vi "Autonomous Independent.vi"() -> ()   [LabVIEW 2012]
doc: "This VI is called when autonomous begins, and will automatically be terminated when autonomous ends. You can carry out timed or sensor driven robot movement independently without needing to return to the caller."
uses:
  <vilib>/Rock Robotics/WPI/SafetyOutput/WPI_SafetyOutputConfigMenu.ctl
  Robot Global Data.vi
  <vilib>/Rock Robotics/WPI/RobotDrive/WPI_RobotDriveGetSetRefNum.vi
  <vilib>/Rock Robotics/WPI/Joystick/WPI_JoystickGetSetRefNum.vi
  <vilib>/Rock Robotics/WPI/RobotDrive/WPI_RobotDriveArcadeDrive_Standard(NoSaturation).vi
panel:
  out "Current Movement, for debugging":T1 {"Y Joystick Value" scale=1.0..-1.0; "X Joystick Value" scale=-1.0..1.0}
  in  "Array of robot movements":T2(array[cluster]) {"Y Joystick Value" scale=1.0..-1.0; "X Joystick Value" scale=-1.0..1.0}
  # "Be sure to right-click and choose Data Operations>>Make Current Value default if you want to save the array values with the VI"
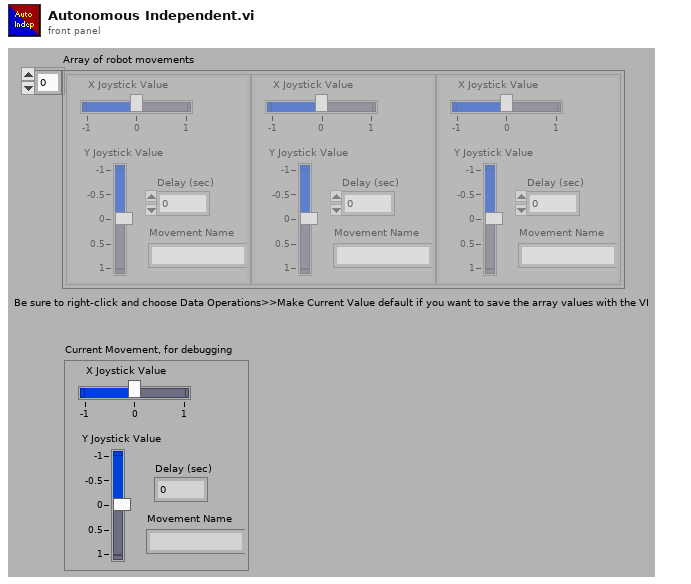
[diagram p1: front panel]
types:
  T1 = cluster{"X Joystick Value":dbl, "Y Joystick Value":dbl, "Delay (sec)":dbl, "Movement Name":string}
  T2 = cluster{"X Joystick Value":dbl, "Y Joystick Value":dbl, "Delay (sec)":dbl, "Movement Name":string}[]
  T3 = typedef "WPI_JoystickDevRef.ctl" = cluster{"Device":T4}
  T4 = typedef "WPI_JoystickDeviceEnum.ctl" = enum16{"USB 1", "USB 2", "USB 3", "USB 4", "Kinect 1", "Kinect 2"}
  T5 = cluster{"axis 1 (x)":dbl, "axis 2 (y)":dbl, "axis 3 (throttle)":dbl, "axis 4":dbl, "axis 5":dbl, "axis 6":dbl}
  T6 = typedef "WPI_SafetyOutputConfigMenu.ctl" = enum16{"Enable", "Disable"}
  T7 = typedef "WPI_RobotDriveDevRef.ctl" = cluster{"DevStatus":errorcluster, "Motors[]":T8[], "Square Inputs":bool, "Max Output":dbl, "Isochronous":bool}
  T8 = typedef "WPI_MotorControlDeviceRef.ctl" = cluster{"DeviceStatus":errorcluster, "Type":enum16{"PWM", "CAN"}, "PWM":cluster{"Digital Module":T9, "PWM Channel":T10, "DeadBand":T11}, "CAN":cluster{"Device Number":u8, "Control Mode":T12, "Semaphore":T13, "Max Vout":dbl}, "Invert":bool, "TransformRef":T14, "InvTransformRef":T14}
  T9 = typedef "FPGA_TypedefDigitalModule.ctl" = enum16{"Digital Module 1", "Digital Module 2"}
  T10 = typedef "FPGA_DIOPWMChannel.ctl" = enum8{"PWM 1", "PWM 2", "PWM 3", "PWM 4", "PWM 5", "PWM 6", "PWM 7", "PWM 8", "PWM 9", "PWM 10", "Invalid"}
  T11 = typedef "WPI_PWMDeadband.ctl" = cluster{"Name":string, "maxPositivePwm":i32, "minPositivePwm":i32, "centerPwm":i32, "maxNegativePwm":i32, "minNegativePwm":i32, "angularRange":u16}
  T12 = typedef "WPI_CANJaguar_ControlMode.ctl" = enum8{"Percent VBus", "Current", "Speed", "Position", "Voltage"}
  T13 = typedef "Semaphore RefNum" = refnum<k1>
  T14 = typedef "WPI_PWMTransform_ConPane.ctl" = refnum<vi>
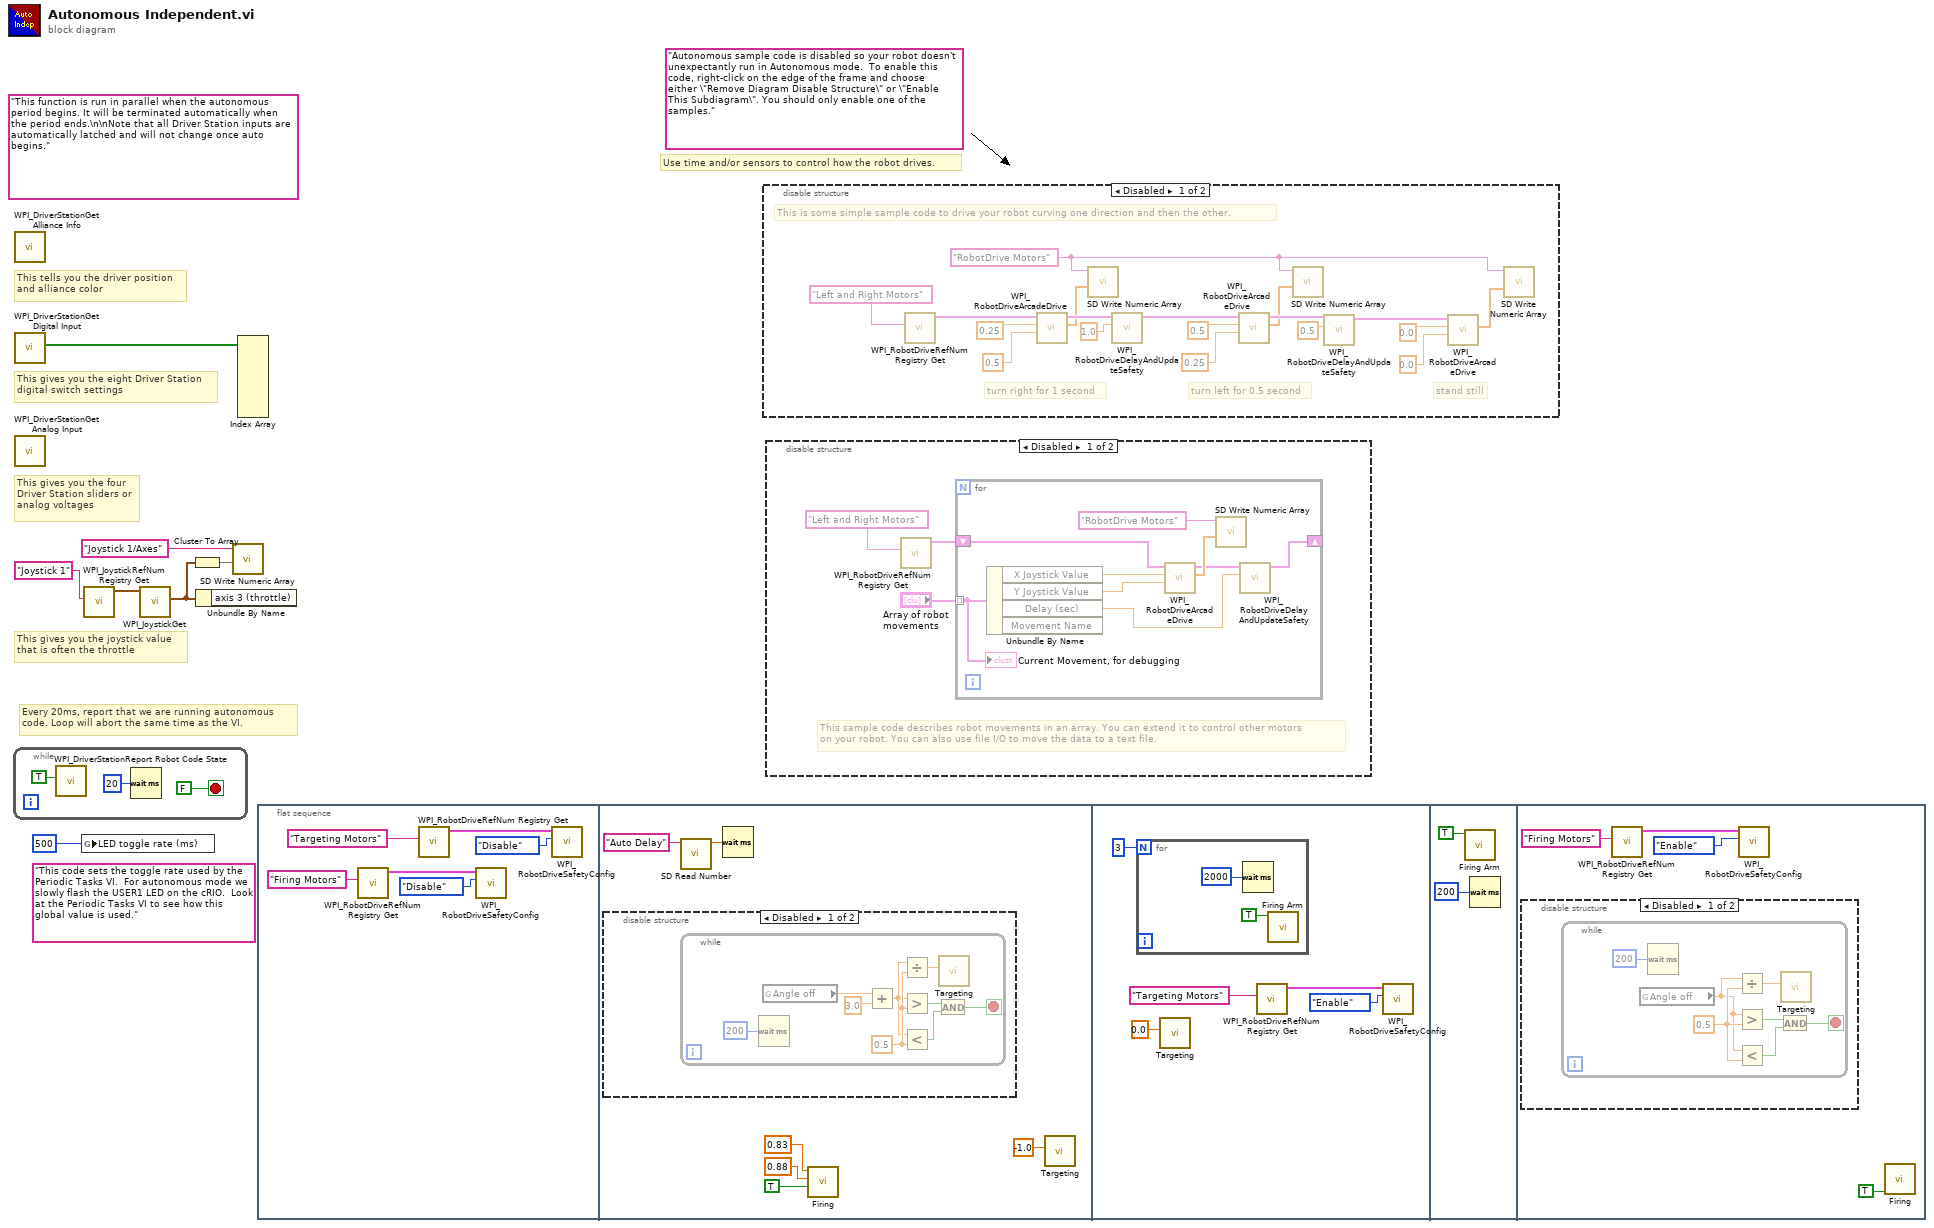
[diagram p0: block diagram]
diagram:
  (unwired) "This code sets the toggle rate used by the Periodic Tasks VI.  For autonomous mode we slowly flash the USER1 LED on the cRIO.  Look at the Periodic Tasks VI to see how this global value is used."
  (unwired) "Autonomous sample code is disabled so your robot doesn't unexpectantly run in Autonomous mode.  To enable this code, right-click on the edge of the frame and choose either \"Remove Diagram Disable Structure\" or \"Enable This Subdiagram\". You should only enable one of the samples."
  (unwired) "This function is run in parallel when the autonomous period begins. It will be terminated automatically when the period ends.\n\nNote that all Driver Station inputs are automatically latched and will not change once auto begins."
  # "Every 20ms, report that we are running autonomous\ncode. Loop will abort the same time as the VI."
  # "This gives you the joystick value\nthat is often the throttle"
  # "Use time and/or sensors to control how the robot drives."
  # "This tells you the driver position\nand alliance color"
  # "This gives you the eight Driver Station\ndigital switch settings"
  # "This gives you the four\nDriver Station sliders or\nanalog voltages"
  n1 = while {
    stop <- FALSE stop-if-true
    n2 = call <vilib>:"WPI_DriverStationReport Robot Code State.vi"("Autonomous"=TRUE) -> ()  [unwired: 10 in, 1 out]
    n3 = Wait (ms)(milliseconds to wait=u32 20) -> ()  [unwired: 1 out]
  }
  n4 = call <vilib>:"WPI_DriverStationGet Alliance Info.vi"() -> ()  [unwired: 12 out]
  n5 = call <vilib>:"WPI_DriverStationGet Digital Input.vi"() -> ("Driver Station Digital Input (1-8)"=w7:bool[])  [unwired: 11 out]
  n6 = call <vilib>:"WPI_DriverStationGet Analog Input.vi"() -> ()  [unwired: 12 out]
  n7 = global write "Robot Global Data.vi" "LED toggle rate (ms)"(u32 500 ("LED ms toggle rate")) -> ()
  n8 = call <vilib>:"WPI_JoystickRefNum Registry Get.vi"("refnum name"="Joystick 1") -> ("JoystickDevRef"=w5:T3)  [unwired: 1 in, 9 out]
  n9 = call <vilib>:"WPI_JoystickGet.vi"("JoystickDevRef"=w5) -> ("Axes"=w2:T5)  [unwired: 1 in, 5 out]
  n10 = Cluster To Array(cluster=w2) -> (array=w3:dbl[])
  n11 = Unbundle By Name(w2) -> ()  [unwired: 1 out]
  n12 = call <vilib>:"SD Write Numeric Array.vi"("Numeric Array"=w3, "Name"="Joystick 1/Axes") -> ()  [unwired: 8 in, 2 out]
  n13 = Index Array(array=w7) -> ()  [unwired: 8 in, 8 out]
  n14 = flat-sequence {
    frame #0 {
      n15 = call <vilib>:"WPI_RobotDriveRefNum Registry Get.vi"("refnum name"="Firing Motors") -> ("RobotDriveDevRef"=w14:T7)  [unwired: 9 in, 1 out]
      n16 = call <vilib>:"WPI_RobotDriveRefNum Registry Get.vi"("refnum name"="Targeting Motors") -> ("RobotDriveDevRef"=w11:T7)  [unwired: 9 in, 1 out]
      n17 = call <vilib>:"WPI_RobotDriveSafetyConfig.vi"("mode"=WPI_SafetyOutputConfigMenu."Disable", "RobotDriveDevRef"=w14) -> ()  [unwired: 8 in, 2 out]
      n18 = call <vilib>:"WPI_RobotDriveSafetyConfig.vi"("mode"=WPI_SafetyOutputConfigMenu."Disable", "RobotDriveDevRef"=w11) -> ()  [unwired: 8 in, 2 out]
    }
    frame #1 {
      n19 = disable-structure shown="Disabled" {
        frame Disabled {
          n20 = while {
            stop <- w31 stop-if-true
            w27 = 0.5 ("y")
            n21 = Wait (ms)(milliseconds to wait=u32 200) -> ()  [unwired: 1 out]
            n22 = global read "Robot Global Data.vi" "Angle off"() -> (w25:dbl)
            n23 = Add(x=w25, y=3.0) -> (x+y=w24:dbl)
            n24 = Divide(x=w24, y=w27) -> (x/y=w28:dbl)
            n25 = Greater?(x=w24, y=w27) -> (0:w30:bool)
            n26 = Less?(x=w24, y=w27) -> (x < y?=w29:bool)
            n27 = And(x=w30, y=w29) -> (x .and. y?=w31:bool)
            n28 = call "Targeting.vi"("Y axis"=w28) -> ()  [unwired: 9 in, 1 out]
          }
        }
        frame Enabled {
        }
      }
      n29 = call <vilib>:"SD Read Number.vi"("Name"="Auto Delay") -> ("Numeric"=w18:dbl)  [unwired: 8 in, 2 out]
      n30 = Wait (ms)(milliseconds to wait=w18) -> ()  [unwired: 1 out]
      n31 = call "Firing.vi"("On"=TRUE, "Speed 2"=0.88, "Speed 1"=0.83) -> ()  [unwired: 6 in, 2 out]
      n32 = call "Targeting.vi"("Y axis"=-1.0) -> ()  [unwired: 9 in, 1 out]
    }
    frame #2 {
      n33 = for {
        N: 3 -> [_]
        n34 = Wait (ms)(milliseconds to wait=u32 2000) -> ()  [unwired: 1 out]
        n35 = call "Firing Arm.vi"("Input"=TRUE) -> ()  [unwired: 11 in]
      }
      n36 = call "Targeting.vi"("Y axis"=0.0) -> ()  [unwired: 9 in, 1 out]
      n37 = call <vilib>:"WPI_RobotDriveRefNum Registry Get.vi"("refnum name"="Targeting Motors") -> ("RobotDriveDevRef"=w34:T7)  [unwired: 9 in, 1 out]
      n38 = call <vilib>:"WPI_RobotDriveSafetyConfig.vi"("mode"=WPI_SafetyOutputConfigMenu."Enable", "RobotDriveDevRef"=w34) -> ()  [unwired: 8 in, 2 out]
    }
    frame #3 {
      n39 = call "Firing Arm.vi"("Input"=TRUE) -> ()  [unwired: 11 in]
      n40 = Wait (ms)(milliseconds to wait=u32 200) -> ()  [unwired: 1 out]
    }
    frame #4 {
      n41 = disable-structure shown="Disabled" {
        frame Disabled {
          n42 = while {
            stop <- w51 stop-if-true
            w47 = 0.5 ("y")
            n43 = global read "Robot Global Data.vi" "Angle off"() -> (w45:dbl)
            n44 = Wait (ms)(milliseconds to wait=u32 200) -> ()  [unwired: 1 out]
            n45 = Divide(x=w45, y=w47) -> (x/y=w48:dbl)
            n46 = Greater?(x=w45, y=w47) -> (0:w50:bool)
            n47 = Less?(x=w45, y=w47) -> (x < y?=w49:bool)
            n48 = And(x=w50, y=w49) -> (x .and. y?=w51:bool)
            n49 = call "Targeting.vi"("Y axis"=w48) -> ()  [unwired: 9 in, 1 out]
          }
        }
        frame Enabled {
        }
      }
      n50 = call <vilib>:"WPI_RobotDriveRefNum Registry Get.vi"("refnum name"="Firing Motors") -> ("RobotDriveDevRef"=w41:T7)  [unwired: 9 in, 1 out]
      n51 = call <vilib>:"WPI_RobotDriveSafetyConfig.vi"("mode"=WPI_SafetyOutputConfigMenu."Enable", "RobotDriveDevRef"=w41) -> ()  [unwired: 8 in, 2 out]
      n52 = call "Firing.vi"("Off"=TRUE) -> ()  [unwired: 8 in, 2 out]
    }
  }
  n53 = disable-structure shown="Disabled" {
    frame Disabled {
      w52 = "RobotDrive Motors" ("Name")
      # "This is some simple sample code to drive your robot curving one direction and then the other."
      # "stand still"
      # "turn left for 0.5 second"
      # "turn right for 1 second"
      n54 = call <vilib>:"WPI_RobotDriveRefNum Registry Get.vi"("refnum name"="Left and Right Motors") -> ("RobotDriveDevRef"=w56:T7)  [unwired: 1 in, 9 out]
      n55 = call-poly <vilib>:"WPI_RobotDriveArcadeDrive.vi"("Y axis value"=0.5 ("X axis value"), "X axis value"=0.25, "RobotDriveDevRef"=w56) -> ("Motor Values"=w55:dbl[], "RobotDriveDevRef"=w63:T7)  [unwired: 1 in, 6 out]
      n56 = call <vilib>:"SD Write Numeric Array.vi"("Numeric Array"=w55, "Name"=w52) -> ()  [unwired: 8 in, 2 out]
      n57 = call <vilib>:"WPI_RobotDriveDelayAndUpdateSafety.vi"("Delay (s)"=1.0, "RobotDriveDevRef"=w63) -> ("RobotDriveDevRef 2"=w62:T7)  [unwired: 8 in, 1 out]
      n58 = call-poly <vilib>:"WPI_RobotDriveArcadeDrive.vi"("Y axis value"=0.25 ("X axis value"), "X axis value"=0.5, "RobotDriveDevRef"=w62) -> ("Motor Values"=w54:dbl[], "RobotDriveDevRef"=w61:T7)  [unwired: 1 in, 6 out]
      n59 = call <vilib>:"SD Write Numeric Array.vi"("Numeric Array"=w54, "Name"=w52) -> ()  [unwired: 8 in, 2 out]
      n60 = call <vilib>:"WPI_RobotDriveDelayAndUpdateSafety.vi"("Delay (s)"=0.5, "RobotDriveDevRef"=w61) -> ("RobotDriveDevRef 2"=w60:T7)  [unwired: 8 in, 1 out]
      n61 = call-poly <vilib>:"WPI_RobotDriveArcadeDrive.vi"("Y axis value"=0.0 ("X axis value"), "X axis value"=0.0, "RobotDriveDevRef"=w60) -> ("Motor Values"=w53:dbl[])  [unwired: 1 in, 7 out]
      n62 = call <vilib>:"SD Write Numeric Array.vi"("Numeric Array"=w53, "Name"=w52) -> ()  [unwired: 8 in, 2 out]
    }
    frame Enabled {
    }
  }
  n63 = disable-structure shown="Disabled" {
    frame Disabled {
      # "This sample code describes robot movements in an array. You can extend it to control other motors\non your robot. You can also use file I/O to move the data to a text file."
      n64 = call <vilib>:"WPI_RobotDriveRefNum Registry Get.vi"("refnum name"="Left and Right Motors") -> ("RobotDriveDevRef"=w71:T7)  [unwired: 1 in, 9 out]
      n65 = for {
        shift-right: [w77] -> _
        shift-left: w71 -> [w78]
        tunnel: "Array of robot movements" -> [w73] mode=indexing
        n66 = Unbundle By Name(w73) -> ("X Joystick Value"=w76:dbl, "Y Joystick Value"=w75:dbl, "Delay (sec)"=w74:dbl)  [unwired: 1 out]
        n67 = call-poly <vilib>:"WPI_RobotDriveArcadeDrive.vi"("Y axis value"=w75, "X axis value"=w76, "RobotDriveDevRef"=w78) -> ("Motor Values"=w80:dbl[], "RobotDriveDevRef"=w79:T7)  [unwired: 1 in, 6 out]
        n68 = call <vilib>:"SD Write Numeric Array.vi"("Numeric Array"=w80, "Name"="RobotDrive Motors") -> ()  [unwired: 8 in, 2 out]
        n69 = call <vilib>:"WPI_RobotDriveDelayAndUpdateSafety.vi"("Delay (s)"=w74, "RobotDriveDevRef"=w79) -> ("RobotDriveDevRef 2"=w77:T7)  [unwired: 8 in, 1 out]
        "Current Movement, for debugging" <- w73
      }
    }
    frame Enabled {
    }
  }
